vi "debugger format results.vi"(8 "error in (no error)":errorcluster, 9 "ENV":T1) -> (0 "error out":errorcluster, 1 "Template Keys":T1)   [LabVIEW 2011]
uses:
  Addons/internet/utils/keyedarr.llb/Keyed Array.ctl
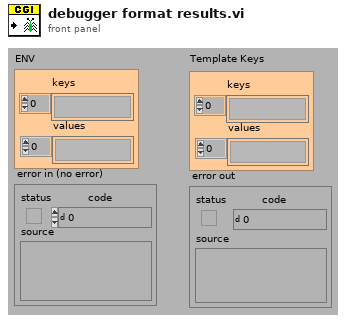
[diagram p1: front panel]
types:
  T1 = typedef "Keyed Array.ctl" = cluster{"keys":string[], "values":string[]}
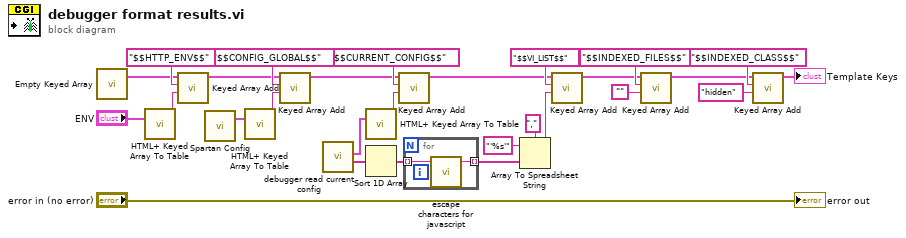
[diagram p0: block diagram]
diagram:
  n1 = call "Empty Keyed Array.vi"() -> ("empty keyed array"=w14:T1)  [unwired: 3 out]
  n2 = call "HTML+ Keyed Array To Table.vi"("keyed array"="ENV") -> ("HTML out"=w21:string)  [unwired: 3 in, 11 out]
  n3 = call "Keyed Array Add.vi"("value"=w21, "key"="$$HTTP_ENV$$", "array in"=w14) -> ("array out"=w13:T1)  [unwired: 2 in, 2 out]
  n4 = call "Spartan Config.vi"() -> ("CONFIG"=w12:T1)  [unwired: 9 in, 2 out]
  n5 = call "HTML+ Keyed Array To Table.vi"("keyed array"=w12) -> ("HTML out"=w19:string)  [unwired: 3 in, 11 out]
  n6 = call "Keyed Array Add.vi"("value"=w19, "key"="$$CONFIG_GLOBAL$$", "array in"=w13) -> ("array out"=w17:T1)  [unwired: 2 in, 2 out]
  n7 = call "debugger read current config.vi"() -> ("VI List"=w9:string[], "Current Config"=w10:T1)  [unwired: 6 in]
  n8 = call "HTML+ Keyed Array To Table.vi"("keyed array"=w10) -> ("HTML out"=w16:string)  [unwired: 3 in, 11 out]
  n9 = Sort 1D Array(array=w9) -> (sorted array=w24:string[])
  n10 = call "Keyed Array Add.vi"("value"=w16, "key"="$$CURRENT_CONFIG$$", "array in"=w17) -> ("array out"=w11:T1)  [unwired: 2 in, 2 out]
  n11 = for {
    tunnel: w24 -> [w29] mode=indexing
    tunnel: [w30] -> w25 mode=indexing
    n12 = call "escape characters for javascript.vi"("String (\"\")"=w29) -> ("escaped String"=w30:string)  [unwired: 4 out]
  }
  n13 = Array To Spreadsheet String(delimiter (Tab)="," ("key"), array=w25, 3:"'%s'" ("key")) -> (spreadsheet string=w28:string)
  n14 = call "Keyed Array Add.vi"("value"=w28, "key"="$$VI_LIST$$", "array in"=w11) -> ("array out"=w6:T1)  [unwired: 2 in, 2 out]
  n15 = call "Keyed Array Add.vi"("value"="", "key"="$$INDEXED_FILES$$", "array in"=w6) -> ("array out"=w3:T1)  [unwired: 2 in, 2 out]
  n16 = call "Keyed Array Add.vi"("value"="hidden" ("key"), "key"="$$INDEXED_CLASS$$", "array in"=w3) -> ("array out"=→"Template Keys":T1)  [unwired: 2 in, 2 out]
  "error out" <- "error in (no error)"
